vi "ExSetupROIThunder.vi"() -> ()   [LabVIEW 2010]
uses:
  Open-Close Hardware/CamHandle.vi
panel:
  out "frames":u32=5341
  out "ADC Speed":u32=20000
  out "error out":errorcluster
  in  "error in (no error)":errorcluster
  in  "Timing Mode":u32(ring)=1 items=["N/A", "Timed Mode/Free run", "Trigger First (only PM)", "Strobed/Ext Sync", "Bulb Mode (PM only)", "Variable Timed mode (PM only)", "Flash Mode (only some PM)"]
  in  "x1":u32=1
  in  "x2":u32=512
  in  "y1":u32=1
  in  "y2":u32=512
  in  "x bin":u32=1
  in  "y bin":u32=1
  in  "min block":u32=2
  in  "Num Min Block":u32=5
  # "ExSetupROI.vi : This vi setups up 1 ROI (Region Of Interest)."
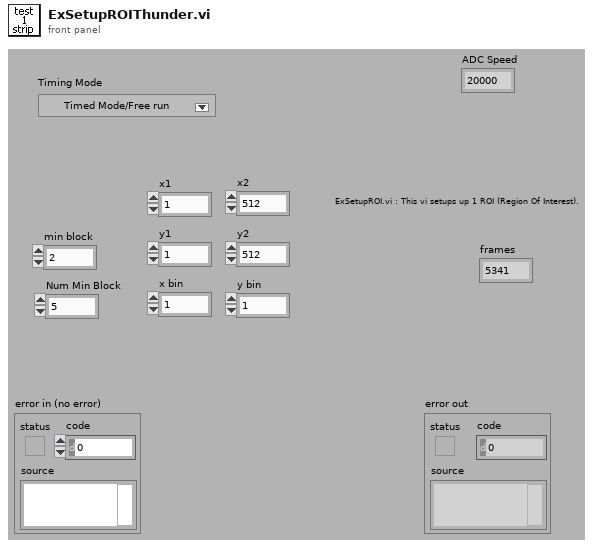
[diagram p1: front panel]
types:
  T1 = cluster{"x1":u32, "x2":u32, "x bin":u32, "y1":u32, "y2":u32, "y bin":u32}
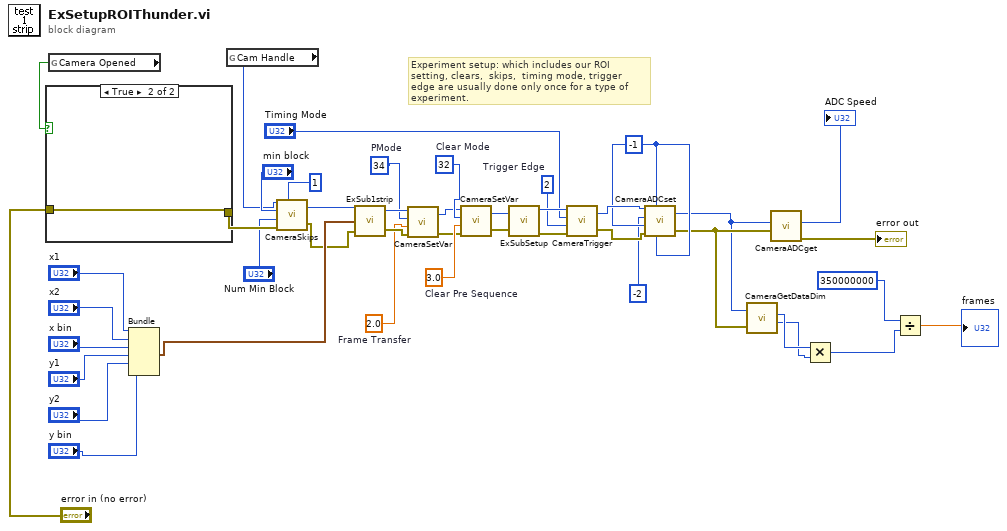
[diagram p0: block diagram]
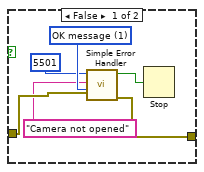
[diagram p2: hidden frame]
diagram:
  w1 = 2.0  # Frame Transfer
  w2 = 34  # PMode
  w7 = 3.0  # Clear Pre Sequence
  w8 = 32  # Clear Mode
  w37 = -1
  w41 = u32 2  # Trigger Edge
  # "Experiment setup: which includes our ROI setting, clears,  skips,  timing mode, trigger edge are usually done only once for a type of experiment."
  n1 = global read "CamHandle.vi" "Camera Opened"() -> (w40:bool)
  n2 = case shown="True" w40 {
    tunnel: "error in (no error)" -> [w48 w50]
    tunnel: [w47 w50] -> w28
    frame False {
      w49 = u16 1 items=["no dialog", "OK message", "continue or stop message"] ("type of dialog (OK msg:1)")
      n3 = call <vilib>:"Simple Error Handler.vi"("error code (no error:0)"=5501, "error source (\" \")"="Camera not opened", "type of dialog (OK msg:1)"=w49, "error in (no error)"=w48) -> ("error?"=w45:bool, "error out"=w47:errorcluster)  [unwired: 1 in, 3 out]
      n4 = Stop(stop? (T)=w45) -> ()
    }
    frame True {
    }
  }
  n5 = Bundle("x1"="x1", "x2"="x2", "x bin"="x bin", "y1"="y1", "y2"="y2", "y bin"="y bin") -> (w29:T1)  [unwired: 1 in]
  n6 = global read "CamHandle.vi" "Cam Handle"() -> (w22:u32)
  n7 = call <userlib>:"CameraSkips.vi"("Camera Handle"=w22, "Minimum Block Size"="min block", "Number of Minimum blocks"="Num Min Block", "error in"=w28, "Type of Skips"=1) -> ("Camera Handle"=w26:u32, "error out"=w27:errorcluster)
  n8 = call "ExSub1strip.vi"("error in (no error)"=w27, "strip 1"=w29, "Camera Handle"=w26) -> ("error out"=w5:errorcluster, "Camera Handle"=w3:u32)
  n9 = call <userlib>:"CameraSetVar.vi"("error in"=w5, "Value"=w1, "Parameter ID"=w2, "Camera Handle"=w3) -> ("error out"=w6:errorcluster, "CameraHandle"=w4:u32)
  n10 = call <userlib>:"CameraSetVar.vi"("error in"=w6, "Value"=w7, "Parameter ID"=w8, "Camera Handle"=w4) -> ("error out"=w11:errorcluster, "CameraHandle"=w10:u32)
  n11 = call "ExSubSetup.vi"("error in (no error)"=w11, "Camera Handle"=w10) -> ("error out"=w42:errorcluster, "Camera Handle"=w43:u32)
  n12 = call <userlib>:"CameraTrigger.vi"("error in"=w42, "Trigger Edge"=w41, "Timing Mode"="Timing Mode", "Camera Handle"=w43) -> ("error out"=w39:errorcluster, "Camera Handle"=w38:u32)
  n13 = call <userlib>:"CameraADCset.vi"("ADC offset"=w37, "Read Out port"=w37, "error in (no error)"=w39, "ADC Gain"=w37, "ADC Speed"=-2, "Camera Handle"=w38) -> ("error out"=w17:errorcluster, "Camera Handle"=w9:u32)
  n14 = call <userlib>:"CameraGetDataDim.vi"("Camera Handle"=w9, "error in"=w17) -> ("Xdim"=w16:u32, "Ydim"=w15:u32)  [unwired: 2 out]
  n15 = call <userlib>:"CameraADCget.vi"("Camera handle"=w9, "error in (no error)"=w17) -> ("ADC Speed"=→"ADC Speed":i32, "error out"=→"error out":errorcluster)  [unwired: 6 out]
  n16 = Multiply(x=w16, y=w15) -> (x*y=w13:u32)
  n17 = Divide(x=350000000, y=w13) -> (x/y=→"frames":dbl)
